vi "Final_Iso.vi"(10 "Array in":dbl[](array[numeric]), 11 "L2T":T1) -> (3 "Array out":bool[](array[boolean]))   [LabVIEW 2020]
uses:
  Ctrl/L2T.ctl
panel:
  # "Pre DCIR_____________________________________"
  # "intra DCIR_____________________________________"
  # "Post DCIR_____________________________________"
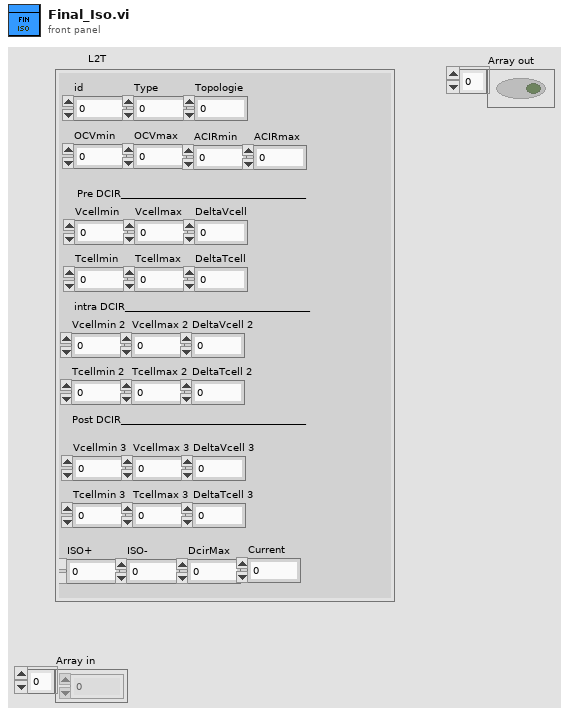
[diagram p1: front panel]
types:
  T1 = typedef "L2T.ctl" = cluster{"id":dbl, "Type":dbl, "OCVmin":dbl, "OCVmax":dbl, "ACIRmin":dbl, "ACIRmax":dbl, "Vcellmin":dbl, "Vcellmax":dbl, "DeltaVcell":dbl, "Tcellmin":dbl, "Tcellmax":dbl, "DeltaTcell":dbl, "ISO+":dbl, "ISO-":dbl, "DcirMax":dbl, "Current":dbl, "Topologie":dbl, "Vcellmin 2":dbl, "Vcellmax 2":dbl, "DeltaVcell 2":dbl, "Tcellmin 2":dbl, "Tcellmax 2":dbl, "DeltaTcell 2":dbl, "Vcellmin 3":dbl, "Vcellmax 3":dbl, "DeltaVcell 3":dbl, "Tcellmin 3":dbl, "Tcellmax 3":dbl, "DeltaTcell 3":dbl}
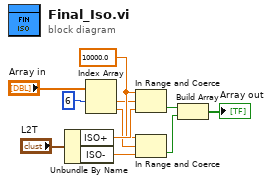
[diagram p0: block diagram]
diagram:
  w7 = 10000.0 ("limite supérieure")
  n1 = Unbundle By Name("L2T") -> ("ISO+"=w11:dbl, "ISO-"=w6:dbl)
  n2 = Index Array(array="Array in", index #1=6 ("index")) -> (element #1=w5:dbl, element #2=w4:dbl)  [unwired: 1 in]
  n3 = In Range and Coerce ("Dans la gamme")(upper limit=w7, x=w5, lower limit=w11) -> (In Range?=w2:bool)  [unwired: 1 out]
  n4 = In Range and Coerce ("Dans la gamme")(upper limit=w7, x=w4, lower limit=w6) -> (In Range?=w3:bool)  [unwired: 1 out]
  n5 = Build Array(w2, w3) -> (→"Array out":bool[])
